vi "Popup.vi"(8 "error in (no error)":errorcluster, 9 "Panel":refnum<class "Panel.lvclass">, 10 "String in":string, 11 "List Data Type in":refnum<class "List Data Type.lvclass">) -> (0 "error out":errorcluster, 2 "String out":string, 3 "List Data Type out":refnum<class "List Data Type.lvclass">)   [LabVIEW 2018, in "List Data Type.lvclass"]
uses:
  List Data Type.lvclass
  <vilib>/MGI/Panel Manager/Panel/Panel/Panel.lvclass
  <vilib>/Utility/miscctls.llb/LVSelectionTypeDef.ctl
  List Data Type.lvclass/List Data Type.ctl
panel:
  in  "Combo Box":string(combo)
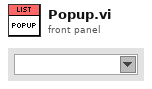
[diagram p1: front panel]
types:
  T1 = typedef "LVSelectionTypeDef.ctl" = cluster{"Selection Start":u32, "Selection End":u32}
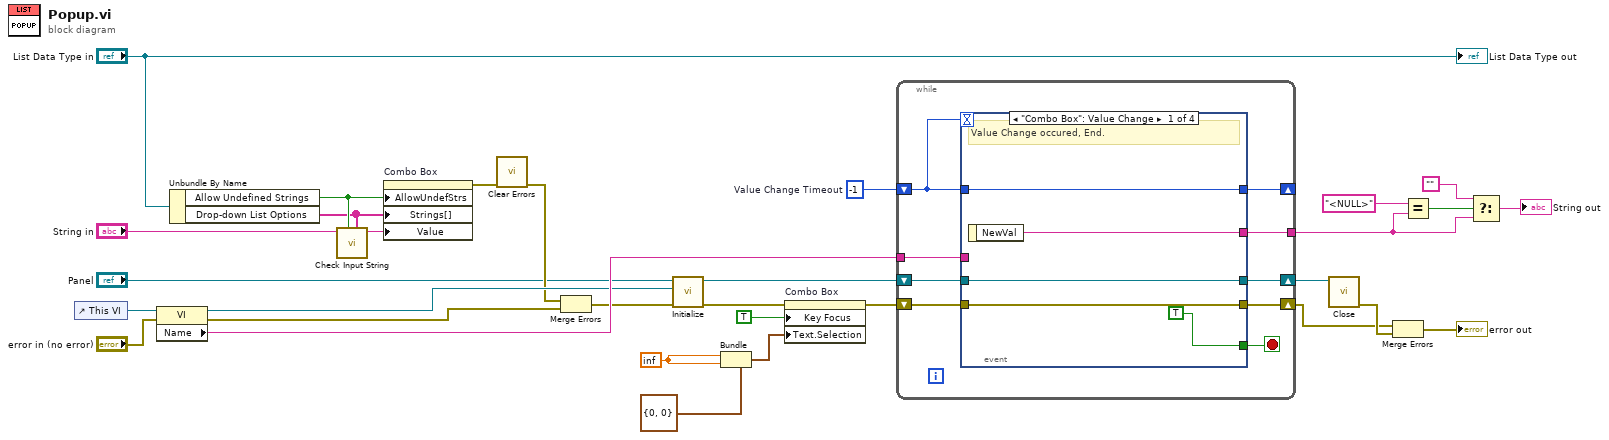
[diagram p0: block diagram]
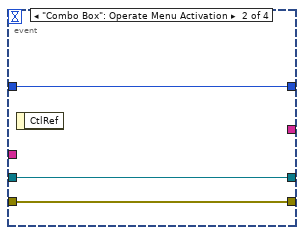
[diagram p2: hidden frame]
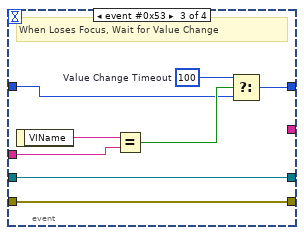
[diagram p3: hidden frame]
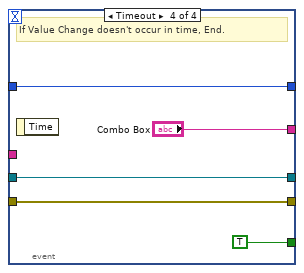
[diagram p4: hidden frame]
diagram:
  w30 = inf
  w25 = -1  # Value Change Timeout
  n1 = control-ref of="This VI"() -> (w20:refnum<vi>)
  n2 = property class="VI"(reference=w20, error in="error in (no error)") -> (reference out=w21:refnum<vi>, error out=w24:errorcluster, "Name"=w23:string)
  n3 = Unbundle By Name("List Data Type in") -> ("Allow Undefined Strings"=w7:bool, "Drop-down List Options"=w6:string[])
  n4 = call "Check Input String.vi"("Drop-down List Options"=w6, "Allow Undefined Strings"=w7, "String in"="String in") -> ("String out"=w8:string)  [unwired: 8 in]
  n5 = property on="Combo Box" class="CmbBox"("AllowUndefStrs"=w7, "Strings[]"=w6, "Value"=w8) -> (error out=w18:errorcluster)  [unwired: 2 in, 1 out]
  n6 = call <vilib>:"Clear Errors.vi"("error in (no error)"=w18) -> ("error out"=w19:errorcluster)  [unwired: 5 in, 1 out]
  n7 = Merge Errors(w19, w24) -> (w22:errorcluster)
  n8 = call <vilib>:"Initialize.vi"("error in (no error)"=w22, "VI Refnum"=w21, "Panel In"="Panel") -> ("error out"=w27:errorcluster, "Panel Out"=w14:refnum<class "Panel.lvclass">)  [unwired: 6 in, 1 out]
  n9 = Bundle(cluster=T1 {"Selection Start"=0, "Selection End"=0} ("Text.Selection"), "Selection Start"=w30, "Selection End"=w30) -> (w31:T1)
  n10 = property on="Combo Box" class="CmbBox"(error in=w27, "Key Focus"=TRUE, "Text.Selection"=w31) -> (error out=w28:errorcluster)  [unwired: 1 in, 1 out]
  n11 = while {
    shift-right: [w40] -> w16
    shift-left: w28 -> [w39]
    shift-right: [w37] -> w15
    shift-left: w14 -> [w36]
    tunnel: [w35] -> w2
    tunnel: w23 -> [w34]
    shift-right: [w32] -> _
    shift-left: w25 -> [w33]
    stop <- w38 stop-if-true
    n12 = event shown="[0] \"Combo Box\": Value Change" {
      selector: _ -> [_ _ _ _]
      dyn-events: _ -> [_ _ _ _]
      timeout: w33 -> [_ _ _ _]
      tunnel: [w42 w46 w54 w59] -> w40
      tunnel: w39 -> [w42 w46 w54 w59]
      tunnel: [TRUE _ _ TRUE] -> w38
      tunnel: [w44 w47 w53 w60] -> w37
      tunnel: w36 -> [w44 w47 w53 w60]
      tunnel: [w43 _ _ "Combo Box"] -> w35
      tunnel: w34 -> [_ _ w55 _]
      tunnel: w33 -> [w41 w48 w50 w57]
      tunnel: [w41 w48 w49 w57] -> w32
      event "Combo Box": Value Change {
        # "Value Change occured, End."
        n13 = event-data() -> ("NewVal"=w43:string)  [unwired: 1 in]
      }
      event "Combo Box": Operate Menu Activation {
        n14 = event-data() -> ()  [unwired: 1 in, 1 out]
      }
      event event #0x53 {
        w51 = 100  # Value Change Timeout
        # "When Loses Focus, Wait for Value Change"
        n15 = event-data() -> ("VIName"=w56:string)  [unwired: 1 in]
        n16 = Equal?(x=w56, y=w55) -> (x = y?=w52:bool)
        n17 = Select(t=w51, s=w52, f=w50) -> (s? t:f=w49:i32)
      }
      event Timeout {
        # "If Value Change doesn't occur in time, End."
        n18 = event-data() -> ()  [unwired: 1 in, 1 out]
      }
    }
  }
  n19 = call-dynamic "Close.vi"("Panel In"=w15) -> ("Error Out"=w17:errorcluster)  [unwired: 10 in]
  n20 = Merge Errors(w16, w17) -> (→"error out":errorcluster)
  n21 = Equal?(x="<NULL>", y=w2) -> (x = y?=w4:bool)
  n22 = Select(t="", s=w4, f=w2) -> (s? t:f=→"String out":string)
  "List Data Type out" <- "List Data Type in"
